vi "Write Server Internal UEs.vi"(8 "error in (no error)":errorcluster, 10 "Server Internal UEs":T1, 11 "SignalGeneratorService in":refnum<class "PluginCore.lvclass">) -> (0 "error out":errorcluster, 3 "SignalGeneratorService out":refnum<class "PluginCore.lvclass">)   [LabVIEW 2021, in "CIF_Plugin_Core_server.lvlib" / "PluginCore.lvclass"]
uses:
  PluginCore.lvclass
  typeDefs/Server Internal UEs.ctl
  typeDefs/Server Internal Message.ctl
  PluginCore.lvclass/PluginCore.ctl
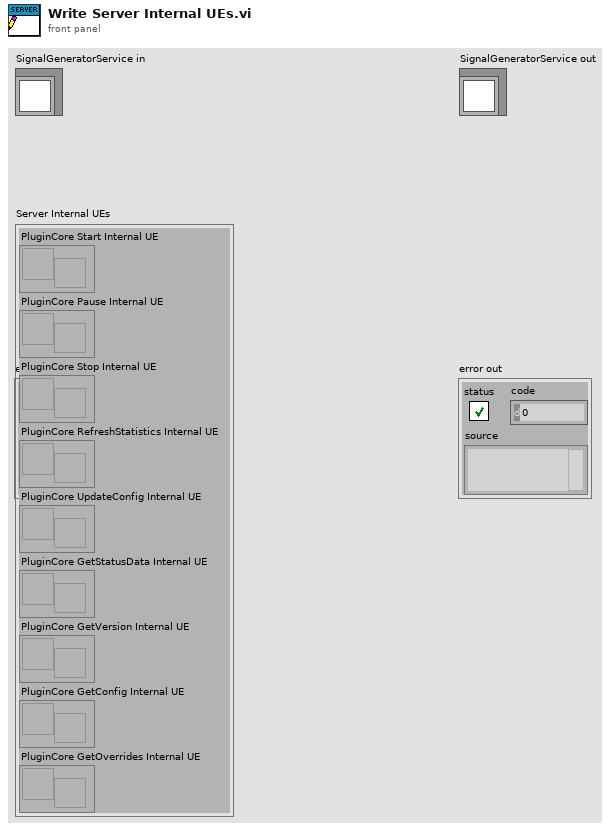
[diagram p1: front panel]
types:
  T1 = typedef "CIF_Plugin_Core_server.lvlib/PluginCore.lvclass/Server Internal UEs.ctl" = cluster{"PluginCore Start Internal UE":refnum<user-event>, "PluginCore Pause Internal UE":refnum<user-event>, "PluginCore Stop Internal UE":refnum<user-event>, "PluginCore RefreshStatistics Internal UE":refnum<user-event>, "PluginCore UpdateConfig Internal UE":refnum<user-event>, "PluginCore GetStatusData Internal UE":refnum<user-event>, "PluginCore GetVersion Internal UE":refnum<user-event>, "PluginCore GetConfig Internal UE":refnum<user-event>, "PluginCore GetOverrides Internal UE":refnum<user-event>}
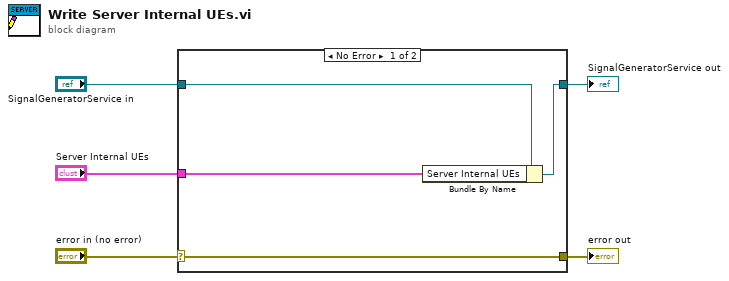
[diagram p0: block diagram]
diagram:
  n1 = case shown="No Error" "error in (no error)" {
    selector: "error in (no error)" -> [w9 w10]
    tunnel: [w9 w10] -> w4
    tunnel: [w7 w11] -> w2
    tunnel: "SignalGeneratorService in" -> [w8 w11]
    tunnel: "Server Internal UEs" -> [w6 _]
    frame No Error {
      n2 = Bundle By Name(cluster=w8, "Server Internal UEs"=w6) -> (w7:refnum<class "PluginCore.lvclass">)
    }
    frame Error {
    }
  }
  "error out" <- w4
  "SignalGeneratorService out" <- w2
